vi "MAIN_merFISH_photobleaching.vi"(4 "error in":errorcluster, 6 "Data cluster":T2, 7 "queue DAQ":refnum<queue>) -> (0 "error out":errorcluster, 3 "Next task":T1)   [LabVIEW 2015]
uses:
  CONTROLS/Q_DAQ_element.ctl
  CONTROLS/Q_main_element.ctl
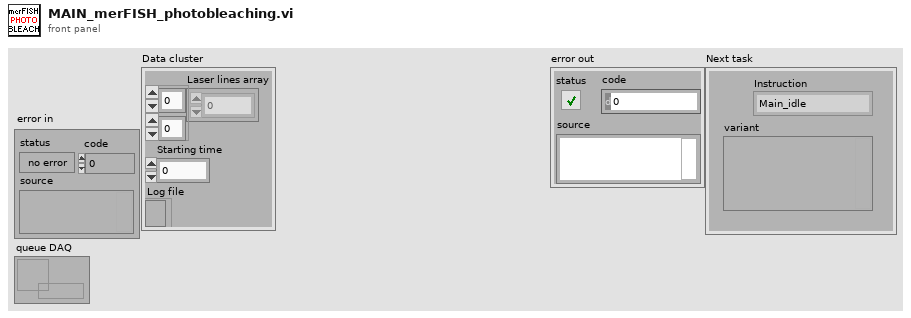
[diagram p1: front panel]
types:
  T1 = typedef "Q_main_element.ctl" = cluster{"variant":variant, "Instruction":enum16{"Main_idle", "Main_initialize", "Main_initialize_TDMS", "Main_initialize_Queue", "Main_error", "Main_DAQ_initialization_results", "Main_ASI_initialization_results", "Main_Piezo_initialization_results", "Main_Valve_initialization_results", "Main_Pump_initialization_results", "Main_CAMERA_initialization_results", "Main_FPGA_initialization_results", "Main_DAQ_error", "Main_ASI_error", "Main_Piezo_error", "Main_CAMERA_error", "Main_Valve_error", "Main_Pump_error", "Main_FPGA_error", "Main_start_acquiring", "Main_not_acquiring", "Main_acquiring", "Main_stop_acquiring", "Main_change_exposure", "Main_change_z_scan_parameters", "Main_define_ROI", "Main_define_mosaic", "Main_read_kinetic_time", "Main_cooler", "Main_read_temperature", "Main_save_XY", "Main_load_XY", "Main_discard_XY", "Main_move_to_XY", "Main_measure_QPD", "Main_autofocus_calibration", "Main_autofocus_initialization", "Main_autofocus_stop", "Main_save_PID", "Main_change_H_valve_position", "Main_two_way_valve", "Main_save_movie", "Main_init_single_scan", "Main_single_scan", "Main_stop_single_scan", "Main_merFISH_illumination_parameters", "Main_merFISH_buffer_probe_list", "Main_merFISH_injections_procedure", "Main_merFISH_save_setpoint", "Main_merFISH_DAPI_parameters", "Main_merFISH_Brightfield_parameters", "Main_merFISH_save_embryo_ROI", "Main_merFISH_init", "Main_merFISH_resume", "Main_merFISH_start_autofocus", "Main_merFISH_open_close_valve_merFISH", "Main_merFISH_open_close_valve_photobleaching", "Main_merFISH_hybridization", "Main_merFISH_move_to_ROI", "Main_merFISH_wait_stabilization", "Main_merFISH_scan", "Main_merFISH_photobleaching_injection", "Main_merFISH_photobleaching", "Main_merFISH_send_email", "Main_merFISH_close", "Main_STOP"}}
  T2 = cluster{"Laser lines array":dbl[][], "Starting time":dbl, "Log file":refnum<file>}
  T3 = typedef "Q_DAQ_element.ctl" = cluster{"variant":variant, "Instruction":enum16{"DAQ_idle", "DAQ_initialize", "DAQ_error", "DAQ_security_stop", "DAQ_init_single_scan", "DAQ_single_scan", "DAQ_init_merFISH", "DAQ_scan_merFISH", "DAQ_photobleaching_merFISH", "DAQ_close_merFISH", "DAQ_stop"}}
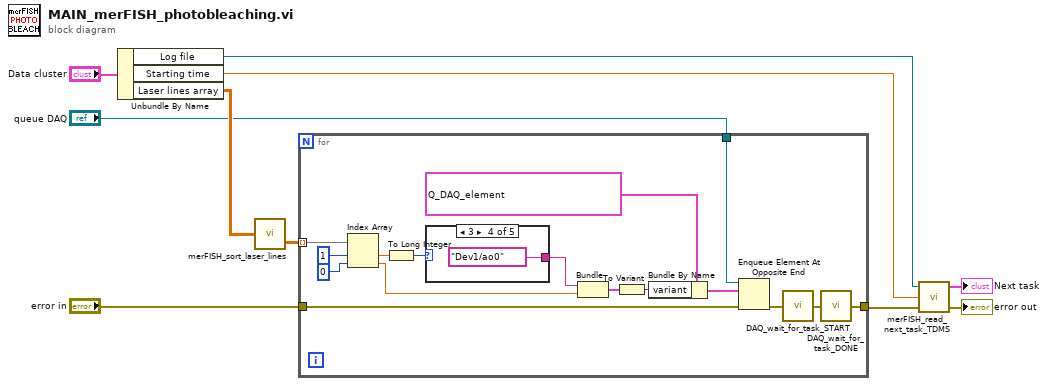
[diagram p0: block diagram]
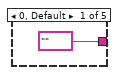
[diagram p2: hidden frame]
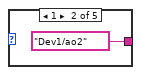
[diagram p3: hidden frame]
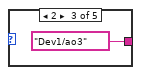
[diagram p4: hidden frame]
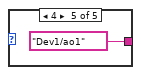
[diagram p5: hidden frame]
diagram:
  n1 = Unbundle By Name("Data cluster") -> ("Log file"=w7:refnum<file>, "Starting time"=w8:dbl, "Laser lines array"=w9:dbl[][])
  n2 = call "merFISH_sort_laser_lines.vi"("Laser lines array"=w9) -> ("Laser lines photobleaching"=w6:dbl[][])  [unwired: 2 in, 2 out]
  n3 = for {
    tunnel: w6 -> [w16] mode=indexing
    tunnel: "error in" -> [w15]
    tunnel: [w13] -> w1
    tunnel: "queue DAQ" -> [w12]
    n4 = Index Array(array=w16, index #1=1 ("index"), index #2=0 ("index")) -> (element #1=w19:dbl, element #2=w21:dbl)
    n5 = To Long Integer(number=w19) -> (32bit integer=w14:i32)
    n6 = case shown="3" w14 {
      tunnel: [tag "" ("Analogic input") tag "Dev1/ao2" ("Analogic input") tag "Dev1/ao3" ("Analogic input") tag "Dev1/ao0" ("Analogic input") tag "Dev1/ao1" ("Analogic input")] -> w20
      frame 0, Default {
      }
      frame 1 {
      }
      frame 2 {
      }
      frame 3 {
      }
      frame 4 {
      }
    }
    n7 = Bundle("Analogic input"=w20, "Laser Power"=w21) -> (w23:cluster{"Analogic input":tag, "Laser Power":dbl})  [unwired: 1 in]
    n8 = To Variant(anything=w23) -> (Variant=w22:variant)
    n9 = Bundle By Name(cluster=T3 {"variant"=variant, "Instruction"=enum."DAQ_photobleaching_merFISH"} ("Q_DAQ"), "variant"=w22) -> (w24:T3)
    n10 = Enqueue Element At Opposite End(queue=w12, element=w24, error in (no error)=w15) -> (error out=w11:errorcluster)  [unwired: 1 in, 2 out]
    n11 = call "DAQ_wait_for_task_START.vi"("error in"=w11) -> ("error out"=w25:errorcluster)
    n12 = call "DAQ_wait_for_task_DONE.vi"("error in"=w25) -> ("error out"=w13:errorcluster)
  }
  n13 = call "merFISH_read_next_task_TDMS.vi"("error in"=w1, "Starting time"=w8, "Log file"=w7) -> ("error out"=→"error out":errorcluster, "task"=→"Next task":T1)  [unwired: 1 in]
